vi "Begin.vi"(8 "error in":errorcluster) -> (0 "error out":errorcluster)   [LabVIEW 2020]
doc: "Called before other user functions, this VI is expected to open initial I/O refnums, load in file data, and do all program initialization. Notice that the <B>error out</B> terminal is simply used for data flow. Wiring it to other structures or subVIs ensures that this VI runs first."
uses:
  <vilib>/Rock Robotics/WPI/DriverStation/WPI_DriverStationRobotMode2.ctl
  <vilib>/Rock Robotics/WPI/Joystick/WPI_JoystickDeviceEnum.ctl
  <vilib>/Rock Robotics/SystemInterfaces/DIO/FPGA_DIOChannel.ctl
  <vilib>/Rock Robotics/SystemInterfaces/spilib/spi_bus.ctl
  Robot Global Data.vi
  <vilib>/Rock Robotics/Network Tables/NT Write String Array.vi
  <vilib>/Rock Robotics/WPI/Switch/WPI_SwitchOpenLimit.vi
  <vilib>/Rock Robotics/WPI/Gyro/WPI_GyroXRS450_SPI_Open.vi
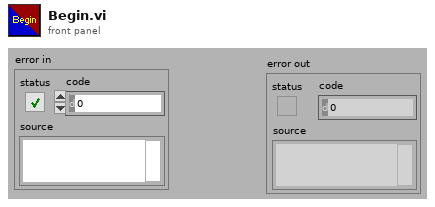
[diagram p1: front panel]
types:
  T1 = typedef "spi_bus.ctl" = enum16{"SPI On-Board, CS0", "SPI On-Board, CS1", "SPI On-Board, CS2", "SPI On-Board, CS3", "SPI MXP", "Invalid"}
  T2 = typedef "FPGA_DIOChannel.ctl" = enum8{"DIO 0", "DIO 1", "DIO 2", "DIO 3", "DIO 4", "DIO 5", "DIO 6", "DIO 7", "DIO 8", "DIO 9", "DIO MXP 0", "DIO MXP 1", "DIO MXP 2", "DIO MXP 3", "DIO MXP 4", "DIO MXP 5", "DIO MXP 6", "DIO MXP 7", "DIO MXP 8", "DIO MXP 9", "DIO MXP 10", "DIO MXP 11", "DIO MXP 12", "DIO MXP 13", "DIO MXP 14", "DIO MXP 15", "SPI Port CS1", "SPI Port CS2", "SPI Port CS3", "SPI Port MISO", "SPI Port MOSI", "Invalid"}
  T3 = typedef "WPI_JoystickDeviceEnum.ctl" = enum16{"USB 0", "USB 1", "USB 2", "USB 3", "USB 4", "USB 5"}
  T4 = typedef "WPI_DriverStationRobotMode2.ctl" = enum16{"Autonomous Disabled", "Autonomous Enabled", "Teleop Disabled", "Teleop Enabled", "Disconnected", "Finish", "Test Disabled", "Test Enabled", "Emergency Stopped"}
  T5 = typedef "WPI_JoystickDevRef.ctl" = cluster{"Device":T3}
  T6 = typedef "WPI_SwitchDevRef.ctl" = cluster{"DevStatus":errorcluster, "DIO Channel":T2, "CntIndex":T7, "Normally Closed":bool}
  T7 = typedef "FPGA_CounterCtrSystemIndex.ctl" = enum8{"Ctr 0", "Ctr 1", "Ctr 2", "Ctr 3", "Ctr 4", "Ctr 5", "Ctr 6", "Ctr 7", "Invalid"}
  T8 = typedef "WPI_GyroDevRef.ctl" = cluster{"DevStatus":errorcluster, "Analog Channel":T9, "Gain (VoltsPerDegree/Second)":dbl, "Gyro Type":enum16{"Analog", "XRS450"}, "Handle":i32, "SPI Bus":T1, "Device Found":bool, "Sample Rate":dbl, "Calibrate On Open":bool, "Offset":dbl}
  T9 = typedef "FPGA_AIChannel.ctl" = enum8{"AI 0", "AI 1", "AI 2", "AI 3", "AI MXP 0", "AI MXP 1", "AI MXP 2", "AI MXP 3", "Invalid"}
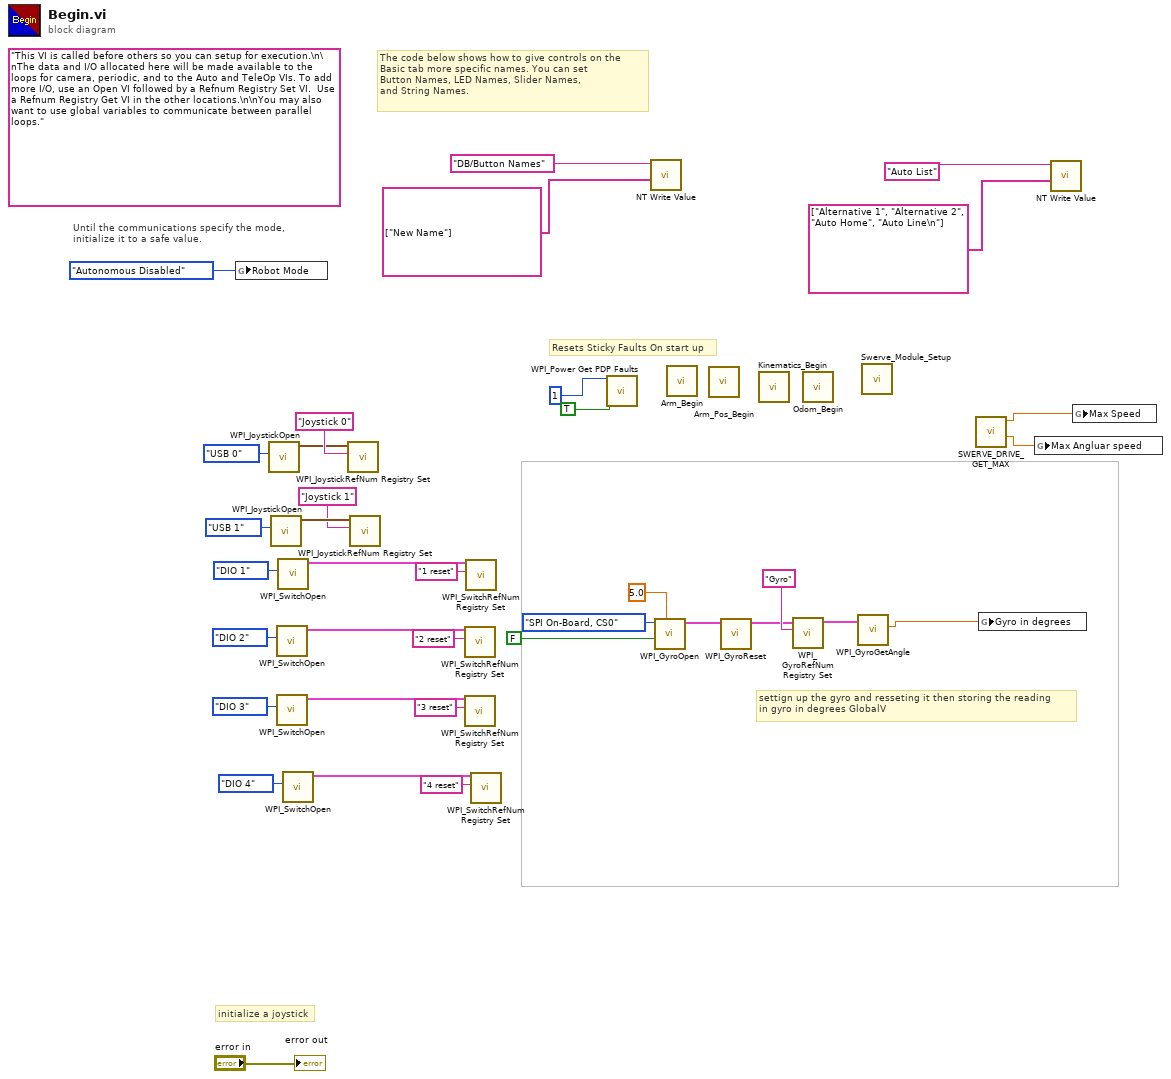
[diagram p0: block diagram]
diagram:
  (unwired) "This VI is called before others so you can setup for execution.\n\nThe data and I/O allocated here will be made available to the loops for camera, periodic, and to the Auto and TeleOp VIs. To add more I/O, use an Open VI followed by a Refnum Registry Set VI.  Use a Refnum Registry Get VI in the other locations.\n\nYou may also want to use global variables to communicate between parallel loops."
  # "Resets Sticky Faults On start up"
  # "settign up the gyro and resseting it then storing the reading \nin gyro in degrees GlobalV"
  # "The code below shows how to give controls on the\nBasic tab more specific names. You can set\nButton Names, LED Names, Slider Names,\nand String Names."
  # "initialize a joystick"
  # "Until the communications specify the mode,\ninitialize it to a safe value."
  n1 = global write "Robot Global Data.vi" "Robot Mode"(WPI_DriverStationRobotMode2."Autonomous Disabled" ("Robot Mode")) -> ()
  n2 = call <vilib>:"WPI_JoystickOpen.vi"("JoystickDevice"=WPI_JoystickDeviceEnum."USB 0") -> ("JoystickDevRef"=w34:T5)  [unwired: 10 in]
  n3 = call <vilib>:"WPI_JoystickOpen.vi"("JoystickDevice"=WPI_JoystickDeviceEnum."USB 1") -> ("JoystickDevRef"=w20:T5)  [unwired: 10 in]
  n4 = call-poly <vilib>:"WPI_SwitchOpen.vi"("DIO Channel"=FPGA_DIOChannel."DIO 2") -> ("SwitchDevRef"=w13:T6)  [unwired: 9 in, 1 out]
  n5 = call-poly <vilib>:"WPI_SwitchOpen.vi"("DIO Channel"=FPGA_DIOChannel."DIO 3") -> ("SwitchDevRef"=w12:T6)  [unwired: 9 in, 1 out]
  n6 = call-poly <vilib>:"WPI_SwitchOpen.vi"("DIO Channel"=FPGA_DIOChannel."DIO 1") -> ("SwitchDevRef"=w18:T6)  [unwired: 9 in, 1 out]
  n7 = call-poly <vilib>:"WPI_SwitchOpen.vi"("DIO Channel"=FPGA_DIOChannel."DIO 4") -> ("SwitchDevRef"=w7:T6)  [unwired: 9 in, 1 out]
  n8 = call <vilib>:"WPI_JoystickRefNum Registry Set.vi"("refnum name"="Joystick 0", "JoystickDevRef"=w34) -> ()  [unwired: 8 in, 2 out]
  n9 = call <vilib>:"WPI_JoystickRefNum Registry Set.vi"("refnum name"="Joystick 1", "JoystickDevRef"=w20) -> ()  [unwired: 8 in, 2 out]
  n10 = call <vilib>:"WPI_SwitchRefNum Registry Set.vi"("refnum name"="2 reset", "SwitchDevRef"=w13) -> ()  [unwired: 8 in, 2 out]
  n11 = call <vilib>:"WPI_SwitchRefNum Registry Set.vi"("refnum name"="3 reset", "SwitchDevRef"=w12) -> ()  [unwired: 8 in, 2 out]
  n12 = call <vilib>:"WPI_SwitchRefNum Registry Set.vi"("refnum name"="1 reset", "SwitchDevRef"=w18) -> ()  [unwired: 8 in, 2 out]
  n13 = call <vilib>:"WPI_SwitchRefNum Registry Set.vi"("refnum name"="4 reset", "SwitchDevRef"=w7) -> ()  [unwired: 8 in, 2 out]
  n14 = call <vilib>:"WPI_Power Get PDP Faults.vi"("Power Distribution (def)"=u8 1, "Clear Sticky Faults"=TRUE) -> ()  [unwired: 9 in, 5 out]
  n15 = call-poly <vilib>:"NT Write Value.vi"("value"=string[] ["New Name"], "name"="DB/Button Names" ("Name")) -> ()  [unwired: 9 in, 1 out]
  n16 = call-poly <vilib>:"WPI_GyroOpen.vi"("Calibration Time (s)"=5.0, "Calibrate On Open"=FALSE, "SPI Bus"=spi_bus."SPI On-Board, CS0") -> ("GyroDevRef"=w23:T8)  [unwired: 6 in, 2 out]
  n17 = call "Arm_Begin.vi"() -> ()  [unwired: 12 in]
  n18 = call "Arm_Pos_Begin.vi"() -> ()  [unwired: 12 in]
  n19 = call <vilib>:"WPI_GyroReset.vi"("GyroDevRef"=w23) -> ("GyroDevRef"=w24:T8)  [unwired: 9 in, 1 out]
  n20 = call "Kinematics_Begin.vi"() -> ()  [unwired: 12 in]
  n21 = call <vilib>:"WPI_GyroRefNum Registry Set.vi"("refnum name"="Gyro", "GyroDevRef"=w24) -> ("GyroDevRef"=w25:T8)  [unwired: 8 in, 1 out]
  n22 = call "Odom_Begin.vi"() -> ()  [unwired: 12 in]
  n23 = call <vilib>:"WPI_GyroGetAngle.vi"("GyroDevRef"=w25) -> ("Angle"=w26:dbl)  [unwired: 6 in, 4 out]
  n24 = call "Swerve_Module_Setup.vi"() -> ()  [unwired: 12 in]
  n25 = call "SWERVE_DRIVE_GET_MAX.vi"() -> ("Max Rotational Vel (Rad/Sec)"=w3:dbl, "Max Wheel Vel (Meter/Sec)"=w4:dbl)  [unwired: 10 in]
  n26 = global write "Robot Global Data.vi" "Gyro in degrees"(w26) -> ()
  n27 = global write "Robot Global Data.vi" "Max Angluar speed"(w3) -> ()
  n28 = call-poly <vilib>:"NT Write Value.vi"("value"=string[] ["Alternative 1", "Alternative 2", "Auto Home", "Auto Line\n"] ("String Array"), "name"="Auto List" ("Name")) -> ()  [unwired: 9 in, 1 out]
  n29 = global write "Robot Global Data.vi" "Max Speed"(w4) -> ()
  "error out" <- "error in"
